vi "AH_CmdSRE.vi"(7 "Tries":i32=5, 8 "error in (no error)":errorcluster, 9 "Arg_1":i32, 10 "Data Cluster In":T1 {"GUI Data Cluster"."SBR" format="%08b"}, 11 "Config Cluster In":T3) -> (0 "error IO":errorcluster, 2 "Data Cluster Out":T1 {"GUI Data Cluster"."SBR" format="%08b"}, 3 "Configuration Cluster Out":T3={"General"={"Config.ini"=path "", "Default Logging Path"=path ""}, "Hardware"={"AHC VISA COM"="", "Measure Rate (1/s)"=0, "Global T VAR"="", "Global B VAR"=""}, "Operation"={"Operation Mode"=enum."Idle-Off", "Status"="", "NewLog?"=FALSE}})   [LabVIEW 2021]
uses:
  Config_Cluster.ctl
  Mode_Enum.ctl
  Data_Cluster.ctl
  Measurement_Cluster.ctl
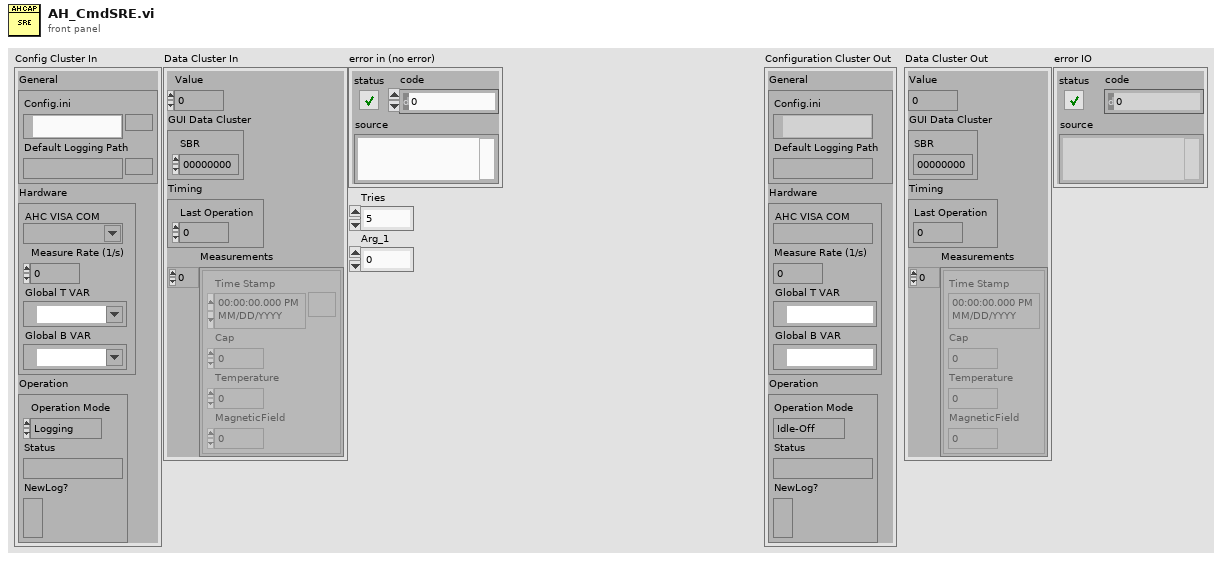
[diagram p1: front panel]
types:
  T1 = typedef "Data_Cluster.ctl" = cluster{"Value":dbl, "GUI Data Cluster":cluster{"SBR":u16}, "Timing":cluster{"Last Operation":dbl}, "Measurements":T2[]}
  T2 = typedef "Measurement_Cluster.ctl" = cluster{"Time Stamp":timestamp, "Cap":dbl, "Temperature":dbl, "MagneticField":dbl}
  T3 = typedef "Config_Cluster.ctl" = cluster{"General":cluster{"Config.ini":path, "Default Logging Path":path}, "Hardware":cluster{"AHC VISA COM":refnum<visa-resource-name>, "Measure Rate (1/s)":i32, "Global T VAR":refnum<k21>, "Global B VAR":refnum<k21>}, "Operation":cluster{"Operation Mode":T4, "Status":string, "NewLog?":bool}}
  T4 = typedef "Mode_Enum.ctl" = enum16{"Logging", "Idle-Off", "Idle"}
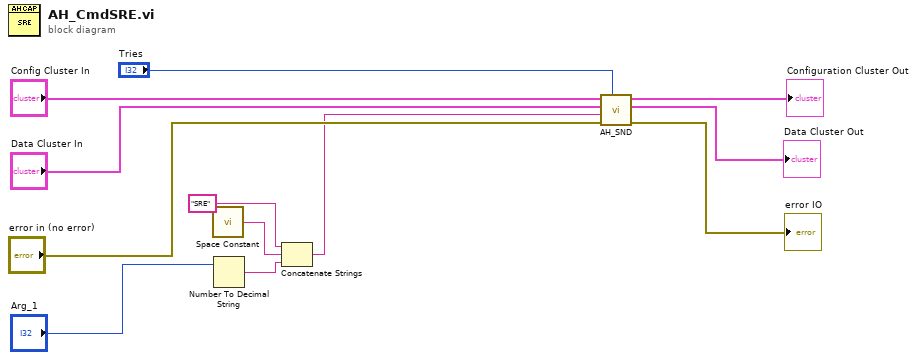
[diagram p0: block diagram]
diagram:
  n1 = call <vilib>:"Space Constant.vi"() -> ("String"=w8:string)
  n2 = Number To Decimal String(number="Arg_1") -> (decimal integer string=w7:string)  [unwired: 1 in]
  n3 = Concatenate Strings("SRE", w8, w7) -> (w4:string)
  n4 = call "AH_SND.vi"("Tries"="Tries", "error in (no error)"="error in (no error)", "CMD"=w4, "Data Cluster In"="Data Cluster In", "Config Cluster In"="Config Cluster In") -> ("error IO"=→"error IO":errorcluster, "Data Cluster Out"=→"Data Cluster Out":T1, "Configuration Cluster Out"=→"Configuration Cluster Out":T3)  [unwired: 4 in]
